vi "SingleJointedArmCtrl_example.vi"() -> ()   [LabVIEW 2019]
uses:
  <vilib>/Rock Robotics/WPI/ThirdParty/JAS_Junk/TrajLib/Trajectory_Library.lvlib
  <vilib>/Analysis/Matrix/Datatypes/RealMatrix.ctl
  <vilib>/Analysis/Matrix/NI_Matrix.lvlib
  <vilib>/Rock Robotics/WPI/ThirdParty/JAS_Junk/TrajLib/TypeDef/LINEAR_SYSTEM.ctl
  <vilib>/Rock Robotics/WPI/ThirdParty/JAS_Junk/TrajLib/TypeDef/DCMOTOR.CTL
  <vilib>/Rock Robotics/WPI/ThirdParty/JAS_Junk/TrajLib/TypeDef/LINEAR_QUADRATIC_REGULATOR.ctl
  <vilib>/Rock Robotics/WPI/ThirdParty/JAS_Junk/TrajLib/TypeDef/KALMAN_FILTER.ctl
  <vilib>/Rock Robotics/WPI/ThirdParty/JAS_Junk/TrajLib/TypeDef/LINEAR_PLANT_INV_FF.ctl
  <vilib>/Rock Robotics/WPI/ThirdParty/JAS_Junk/TrajLib/TypeDef/LINEAR_SYSTEM_LOOP.ctl
  <vilib>/Rock Robotics/WPI/ThirdParty/JAS_Junk/TrajLib/TypeDef/LINEAR_SYSTEM_SIM.ctl
  <vilib>/Rock Robotics/WPI/ThirdParty/JAS_Junk/TrajLib/TypeDef/SINGLE_JOINT_ARM_SIM.ctl
panel:
  in  "Tab Control":T1(tab)
  in  "SP 4":bool
  in  "SP 3":bool
  in  "SP 2":bool
  in  "SP 1":bool
  out "Battery Voltage":dbl format="%20.3f"
  out "CO Chart":T2(graph)
  in  "SP 0":bool
  out "Arm Position\nDegrees":dbl(knob) scale=0.0..180.0
  out "Process Variable \nDegrees":dbl format="%17.1f"
  out "Kalman Filtered\nArm Angle":dbl format="%17.1f"
  out "PV Chart":T3(graph)
  out "Error":bool
  out "Motor Volt Dmd (CO)":dbl format="%20.3f"
  out "At Top":bool
  out "At Bottom":bool
  out "Motor Amps":dbl format="%20.3f"
  out "Setpoint Degrees":dbl format="%17.1f"
  out "Arm Motor":T4 {"Jr_KgM2" format="%13.5p"; "L_H" format="%13.5p"; "Kt_NMPerAmp" format="%13.5p"; "KvINV_RadPerSecPerVolt" format="%13.5p"; "R_Ohms" format="%13.5p"; "FreeSpeed_RadPerSec" format="%13.5p"; "FreeCurrent_Amps" format="%13.5p"; "StallCurrent_Amps" format="%13.5p"; "StallTorque_NM" format="%13.5p"; "nominalVoltage_Volts" format="%13.5p"}
  out "m_Arm":T5
  out "Single Joint Arm Simulaation":T7 {"GearBox"."Jr_KgM2" format="%13.5p"; "GearBox"."L_H" format="%13.5p"; "GearBox"."Kt_NMPerAmp" format="%13.5p"; "GearBox"."KvINV_RadPerSecPerVolt" format="%13.5p"; "GearBox"."R_Ohms" format="%13.5p"; "GearBox"."FreeSpeed_RadPerSec" format="%13.5p"; "GearBox"."FreeCurrent_Amps" format="%13.5p"; "GearBox"."StallCurrent_Amps" format="%13.5p"; "GearBox"."StallTorque_NM" format="%13.5p"; "GearBox"."nominalVoltage_Volts" format="%13.5p"}
  out "KalmanFilter":T9
  out "Kalman Error":errorcluster
  out "LinearQuadraticRegulator":T10
  out "LQR Error":bool
  out "Linear System Loop":T11
  out "LinSysLoop_Error":bool
  # "Set Position\nDemand"
  # "Single Jointed Arm Simulation"
  # "<States,States>"
  # "<States,Inputs>"
  # "<Outputs,States>"
  # "<Outputs,Inputs>"
  # "<States, 1>"
  # "<Outputs, 1>"
  # "<Inputs, 1>"
  # "<Outputs, 1>"
  # "<States,States>"
  # "<States,Inputs>"
  # "<Outputs,States>"
  # "<Outputs,Inputs>"
  # "Steady State Gain  \n<States,Outputs>"
  # "State Estimate <Statess,1>"
  # "<States,States>"
  # "<States,Inputs>"
  # "<Outputs,States>"
  # "<Outputs,Inputs>"
  # "Ref State <States,1>"
  # "Comp and capped \noutput <Inputs,1>"
  # "Controller gain\n<Inputs,States>"
  # "<States,1>"
  # "<FUTURE --- CLAMP TYPE -- For now\nuse Normalize>"
  # "Steady State Gain  \n<States,Outputs>"
  # "State Estimate <Statess,1>"
  # "<States,States>"
  # "<States,Inputs>"
  # "<Outputs,States>"
  # "<Outputs,Inputs>"
  # "<States,1>"
  # "<Inputs,1>"
  # "<States,Inputs>"
  # "<States,States>"
  # "Ref State <States,1>"
  # "Comp and capped \noutput <Inputs,1>"
  # "Controller gain\n<Inputs,States>"
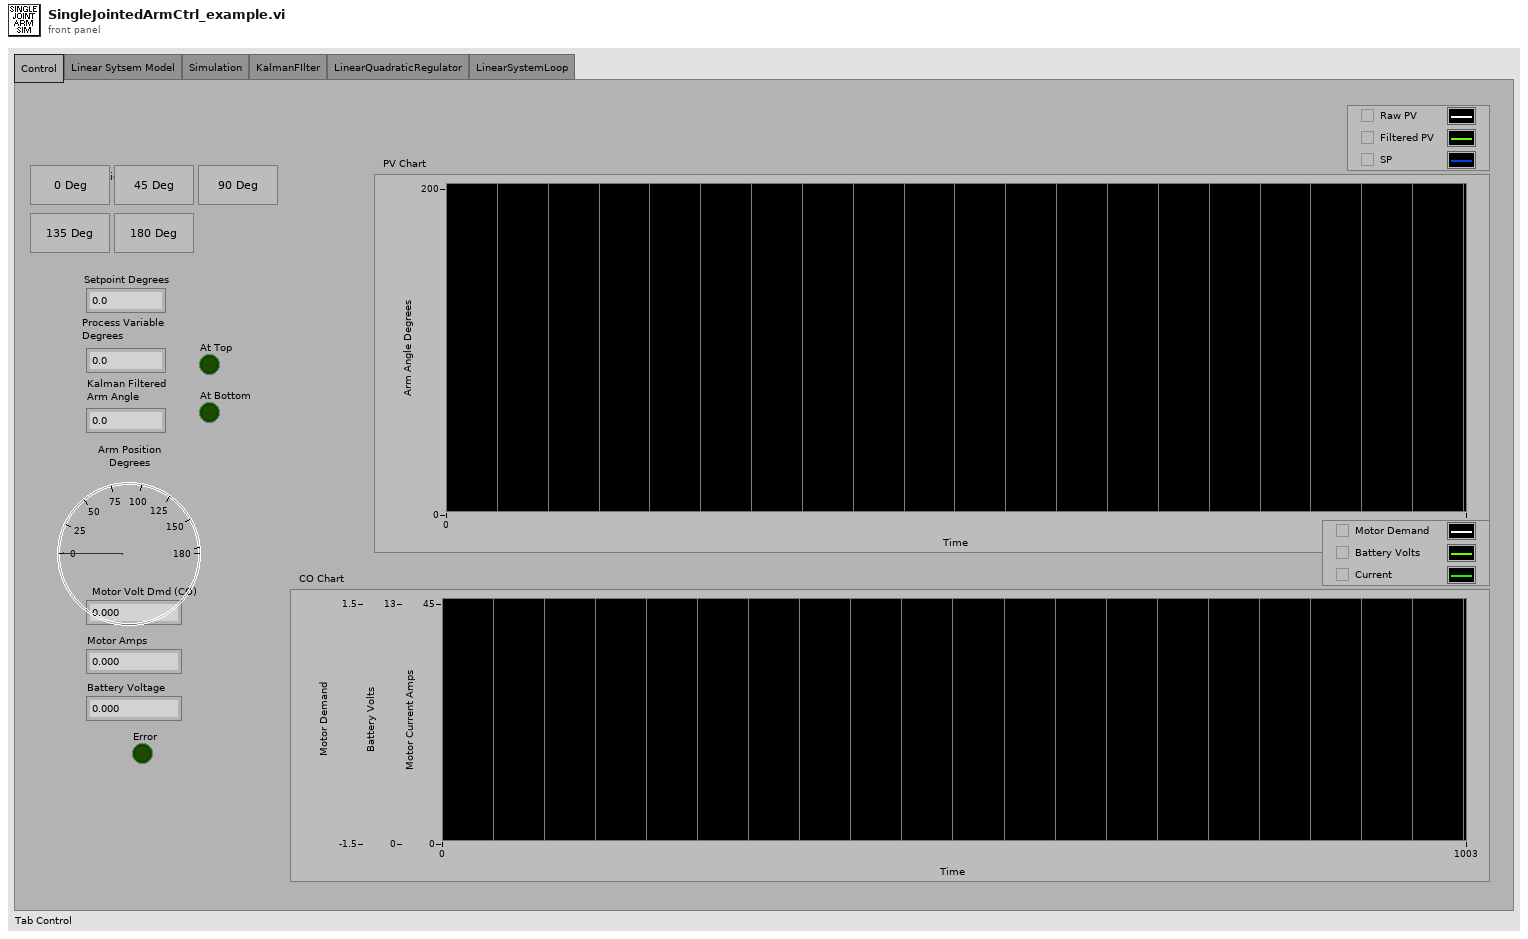
[diagram p1: front panel]
types:
  T1 = enum32{"Control", "Linear Sytsem Model", "Simulation", "KalmanFIlter", "LinearQuadraticRegulator", "LinearSystemLoop"}
  T2 = cluster{"Motor Dmd":dbl, "Voltage":dbl, "Motor Current":dbl}
  T3 = cluster{"upper limit":dbl, "Real Matrix Element":dbl, "Real Matrix Element":dbl}
  T4 = typedef "Trajectory_Library.lvlib/DCMOTOR.CTL" = cluster{"nominalVoltage_Volts":dbl, "StallTorque_NM":dbl, "StallCurrent_Amps":dbl, "FreeCurrent_Amps":dbl, "FreeSpeed_RadPerSec":dbl, "R_Ohms":dbl, "KvINV_RadPerSecPerVolt":dbl, "Kt_NMPerAmp":dbl, "L_H":dbl, "Jr_KgM2":dbl}
  T5 = typedef "Trajectory_Library.lvlib/LINEAR_SYSTEM.ctl" = cluster{"m_A":T6, "m_B":T6, "m_C":T6, "m_D":T6, "States":i32, "Inputs":i32, "Outputs":i32}
  T6 = typedef "NI_Matrix.lvlib/RealMatrix.ctl" = dbl[][]
  T7 = typedef "Trajectory_Library.lvlib/SINGLE_JOINT_ARM_SIM.ctl" = cluster{"Arm_LinearSystem":T8, "GearBox":T4, "Gearing":dbl, "R_ArmLength_M":dbl, "MinAngle_Rad":dbl, "MaxAngle_Rad":dbl, "SimulateGravity":bool}
  T8 = typedef "Trajectory_Library.lvlib/LINEAR_SYSTEM_SIM.ctl" = cluster{"m_Plant":T5, "m_X":T6, "m_Y":T6, "m_U":T6, "MeasureStdDev":T6}
  T9 = typedef "Trajectory_Library.lvlib/KALMAN_FILTER.ctl" = cluster{"m_K":T6, "m_xHat":T6, "States":i32, "Outputs":i32, "m_Plant":T5}
  T10 = typedef "Trajectory_Library.lvlib/LINEAR_QUADRATIC_REGULATOR.ctl" = cluster{"m_r":T6, "m_U":T6, "m_K":T6, "States":i32, "Inputs":i32}
  T11 = typedef "Trajectory_Library.lvlib/LINEAR_SYSTEM_LOOP.ctl" = cluster{"Controller":T10, "FeedForward":T12, "Observer":T9, "Next_R":T6, "Clamp Max":T6}
  T12 = typedef "Trajectory_Library.lvlib/LINEAR_PLANT_INV_FF.ctl" = cluster{"m_R":T6, "m_Uff":T6, "m_B":T6, "m_A":T6, "States":i32, "Inputs":i32}
  T13 = cluster{"Degrees":dbl, "Degrees":dbl, "Degrees":dbl}
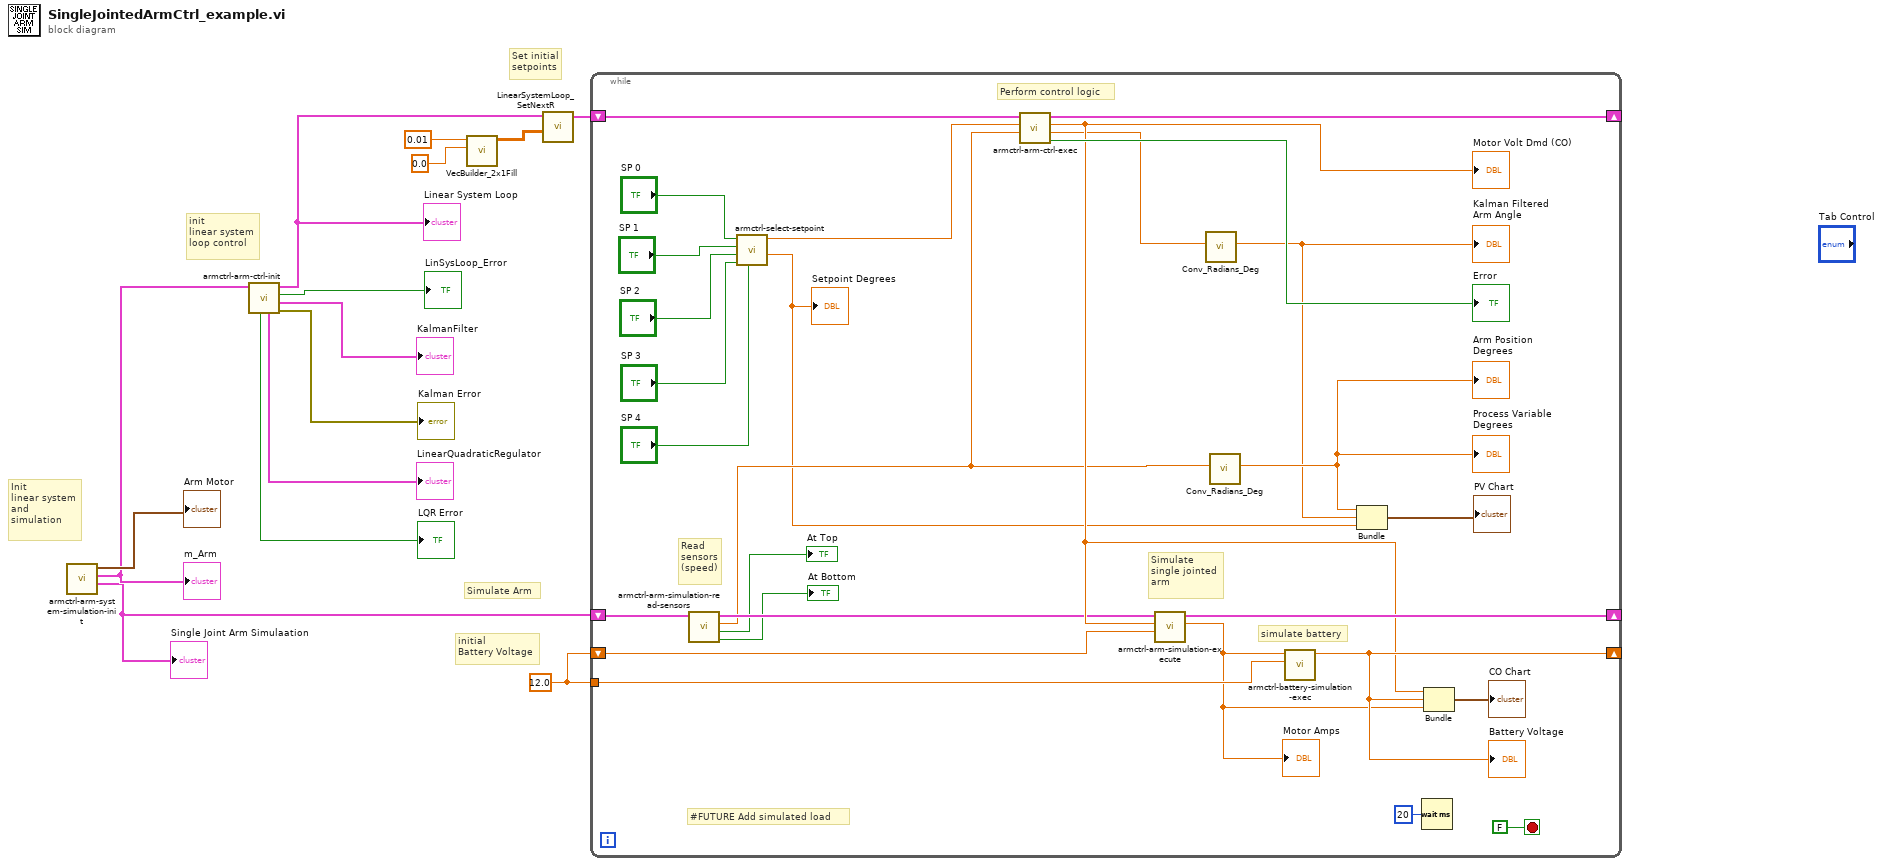
[diagram p0: block diagram]
diagram:
  w13 = 12.0
  # "Set initial\nsetpoints"
  # "init\nlinear system\nloop control"
  # "Init\nlinear system\nand \nsimulation"
  # "Simulate Arm"
  # "initial\nBattery Voltage"
  n1 = call "armctrl-arm-system-simulation-init.vi"() -> ("SingleJointArmSim"=w1:T7, "Linearsystem"=w8:T5, "DCMOTOR"=→"Arm Motor":T4)  [unwired: 9 in]
  "m_Arm" <- w8
  "Single Joint Arm Simulaation" <- w1
  n2 = call "armctrl-arm-ctrl-init.vi"("Linearsystem"=w8) -> ("Kalman Error"=→"Kalman Error":errorcluster, "KalmanFilter"=→"KalmanFilter":T9, "LinSysLoopError"=→"LinSysLoop_Error":bool, "Linear System Loop"=w2:T11, "LinearQuadraticRegulator"=→"LinearQuadraticRegulator":T10, "Lqr Error"=→"LQR Error":bool)  [unwired: 5 in]
  "Linear System Loop" <- w2
  n3 = call <vilib>:"VecBuilder_2x1Fill.vi"("R1"=0.0, "R0"=0.01 ("R0_C0")) -> ("output matrix"=w9:T6)  [unwired: 9 in]
  n4 = call <vilib>:"LinearSystemLoop_SetNextR.vi"("R"=w9, "input inear System Loop"=w2) -> ("out Linear System Loop"=w11:T11)  [unwired: 8 in, 1 out]
  n5 = while {
    shift-right: [w37] -> _
    shift-left: w11 -> [w34]
    shift-right: [w36] -> _
    shift-left: w1 -> [w25]
    shift-right: [w38] -> _
    shift-left: w13 -> [w26]
    tunnel: w13 -> [w35]
    stop <- FALSE stop-if-true
    # "simulate battery"
    # "Simulate\nsingle jointed\narm"
    # "Perform control logic"
    # "Read\nsensors\n(speed)"
    # "#FUTURE Add simulated load"
    n6 = call "armctrl-arm-simulation-read-sensors.vi"("SingleJointArmSim"=w25) -> ("AtLowLimit"=→"At Bottom":bool, "At HIgh LImit"=→"At Top":bool, "ArmAngle_Rad"=w21:dbl, "out SingleJointArmSim"=w22:T7)  [unwired: 7 in]
    n7 = call "armctrl-select-setpoint.vi"("Set 180"="SP 4", "Set 135"="SP 3", "Set 90"="SP 2", "Set 45"="SP 1", "Set 0"="SP 0") -> ("Degrees"=w15:dbl, "Radians"=w28:dbl)  [unwired: 4 in, 1 out]
    "Setpoint Degrees" <- w15
    n8 = call "armctrl-arm-ctrl-exec.vi"("Process Variable\nRadians"=w21, "Setpoint Radians"=w28, "in Linear System Loop"=w34) -> ("Error"=→"Error":bool, "Filtered Process\nVariable Radians"=w17:dbl, "Motor Dmd"=w23:dbl, "out Linear System Loop"=w37:T11)  [unwired: 5 in]
    "Motor Volt Dmd (CO)" <- w23
    n9 = call "armctrl-arm-simulation-execute.vi"("Battery Volts"=w26, "Motor Dmd"=w23, "in SingleJointArmSim"=w22) -> ("Motor Current"=w24:dbl, "out SingleJointArmSim"=w36:T7)  [unwired: 7 in]
    "Motor Amps" <- w24
    n10 = call <vilib>:"Conv_Radians_Deg.vi"("Radians"=w17) -> ("Degrees"=w16:dbl)  [unwired: 10 in]
    "Kalman Filtered\nArm Angle" <- w16
    n11 = call <vilib>:"Conv_Radians_Deg.vi"("Radians"=w21) -> ("Degrees"=w18:dbl)  [unwired: 10 in]
    "Arm Position\nDegrees" <- w18
    "Process Variable \nDegrees" <- w18
    n12 = call "armctrl-battery-simulation-exec.vi"("Numeric"=w35, "Motor Current"=w24) -> ("Voltage"=w38:dbl)  [unwired: 9 in]
    "Battery Voltage" <- w38
    n13 = Bundle("Degrees"=w18, "Degrees"=w16, "Degrees"=w15) -> (→"PV Chart":T13)  [unwired: 1 in]
    n14 = Wait (ms)(milliseconds to wait=u32 20) -> ()  [unwired: 1 out]
    n15 = Bundle("Motor Dmd"=w23, "Voltage"=w38, "Motor Current"=w24) -> (→"CO Chart":T2)  [unwired: 1 in]
  }
